vi "Shared Variable Server.vi"() -> ()   [LabVIEW 2017]
doc: "This VI hosts two shared variables that can be accessed by a variety of client VIs. Shared Variables are typically used for monitoring lossy data, like memory usage, temperature data, etc."
panel:
  in  "Stop":bool
  # "Overview: Demonstrates the use of Network-Published Shared Variables to provide monitoring data to a variety of client VIs.\nRequirements: Windows\nInstructions:\n1. Run this VI.\n2. Run each of the Shared Variable Client VIs in the project to see the different ways you can connect to shared variables. Note that any number of client VIs can run at the same time.\n3. Once you have stopped all the client VIs, click Stop to stop this VI."
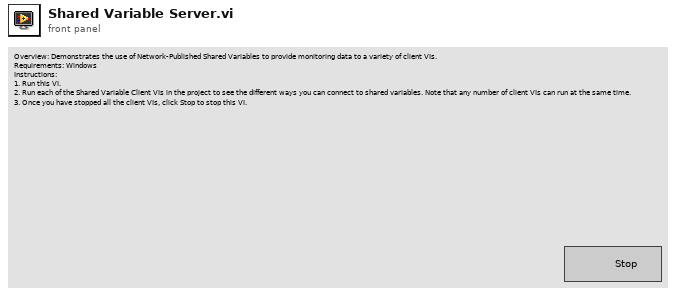
[diagram p1: front panel]
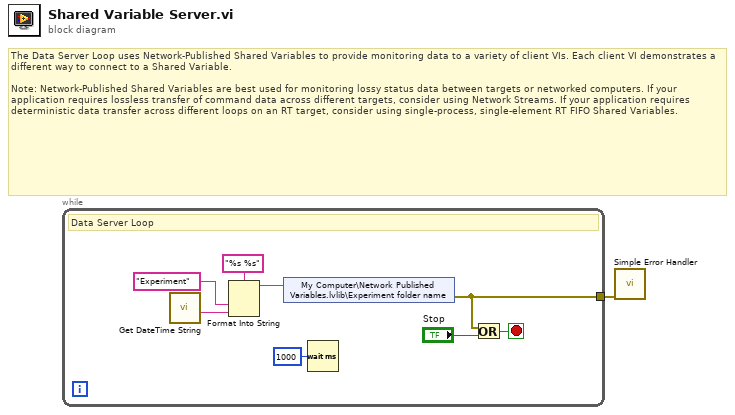
[diagram p0: block diagram]
diagram:
  # "The Data Server Loop uses Network-Published Shared Variables to provide monitoring data to a variety of client VIs. Each client VI demonstrates a different way to connect to a Shared Variable.\n\nNote: Network-Published Shared Variables are best used for monitoring lossy status data between targets or networked computers. If your application requires lossless transfer of command data across different targets, consider using Network Streams. If your application requires deterministic data transfer across different loops on an RT target, consider using single-process, single-element RT FIFO Shared Variables."
  n1 = while {
    tunnel: [w6] -> w1
    stop <- w8 stop-if-true
    # "Data Server Loop"
    n2 = call <userlib>:"Get DateTime String.vi"() -> ("Time string"=w5:string)  [unwired: 10 in, 1 out]
    n3 = Format Into String(format string="%s %s", "Experiment" ("input 1"), w5) -> (resulting string=w2:string)  [unwired: 2 in, 1 out]
    n4 = shared-variable "My Computer\\Network Published Variables.lvlib\\Experiment folder name"(w2) -> (error out=w6:errorcluster)  [unwired: 1 in]
    n5 = Wait (ms)(milliseconds to wait=u32 1000) -> ()  [unwired: 1 out]
    n6 = Or(x=w6, y="Stop") -> (x .or. y?=w8:bool)
  }
  n7 = call <vilib>:"Simple Error Handler.vi"("error in (no error)"=w1) -> ()  [unwired: 4 in, 5 out]
